vi "BGK Data Acquisition Loop - NLHQ.vi"(7 "Period (s)":dbl=600.0 caption="采样周期 (s)" format="%#_13g", 8 "error in (no error)":errorcluster caption="错误输入（无错误）", 11 "Message Queues":T1 caption="消息队列") -> (0 "error out":errorcluster caption="错误输出")   [LabVIEW 2015]
uses:
  Support VIs/Message Queue/All Real-Time Message Queues.ctl
  Support VIs/Message Queue/Message Cluster.ctl
  <vilib>/Platform/TimedLoop/XDataNode/timing_clust.ctl
  <vilib>/Platform/TimedLoop/XDataNode/nitl_modes.ctl
  <vilib>/Platform/TimedLoop/XDataNode/wakeup.ctl
  <vilib>/Instr/_visa.llb/VISA Configure Serial Port (Instr).vi
  Globals/Global - Monitoring Variables.vi
  <vilib>/Platform/TimedLoop/XDataNode/loadnilvce.vi
  Globals/Global - All RT Loop Stop.vi
  <vilib>/Platform/TimedLoop/XDataNode/XDataNode.xnode
  <vilib>/Platform/TimedLoop/XDataNode/XDNodeRunTimeDep.lvlib
  Support VIs/Message Queue/Message Queue.lvlib
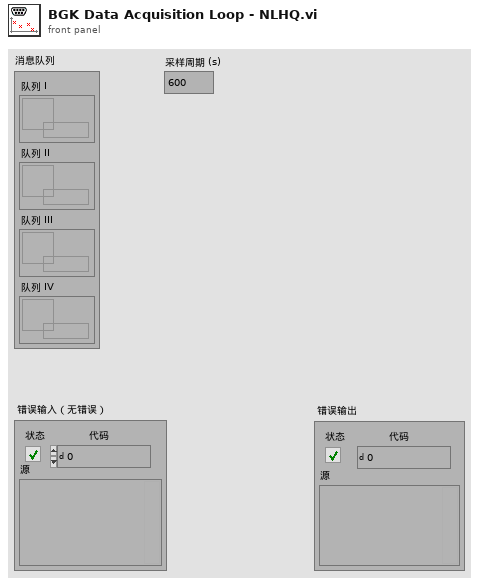
[diagram p1: front panel]
types:
  T1 = typedef "Message Queue.lvlib/All Real-Time Message Queues.ctl" = cluster{"Queue I":refnum<queue>, "Queue II":refnum<queue>, "Queue III":refnum<queue>, "Queue IV":refnum<queue>}
  T2 = typedef "XDNodeRunTimeDep.lvlib/timing_clust.ctl" = cluster{"Expected End [f-1]":u64, "Actual End [f-1]":u64, "Finished Late? [f-1]":bool, "Expected End [i-1]":u64, "Actual End [i-1]":u64, "Finished Late? [i-1]":bool, "Expected Start [i]":u64, "Actual Start [i]":u64, "Expected Start [f]":u64, "Actual Start [f]":u64, "Source Name":string, "Structure Name":string, "Period":i64, "Deadline":i64, "Offset":i64, "Start":i64, "Priority":i32, "Timeout":i32, "Mode":T3, "Wakeup Reason":T4, "Error":errorcluster, "Source Type":string, "Secondary Source Type":string, "Global End Time":u64, "Global Start Time":u64, "Frame Duration":u64, "Iteration Duration":u64, "Assigned CPU":i32, "I/O Scan Engine Mode":u32}
  T3 = typedef "XDNodeRunTimeDep.lvlib/nitl_modes.ctl" = enum32{"No Change", "Process missed periods, maintain original phase", "Discard missed periods, maintain original phase", "Process missed periods, ignore original phase", "Discard missed periods, ignore original phase"}
  T4 = typedef "XDNodeRunTimeDep.lvlib/wakeup.ctl" = enum32{"Normal", "Aborted", "Asynchronous wakeup", "Timing source error", "Timed loop error", "Timeout"}
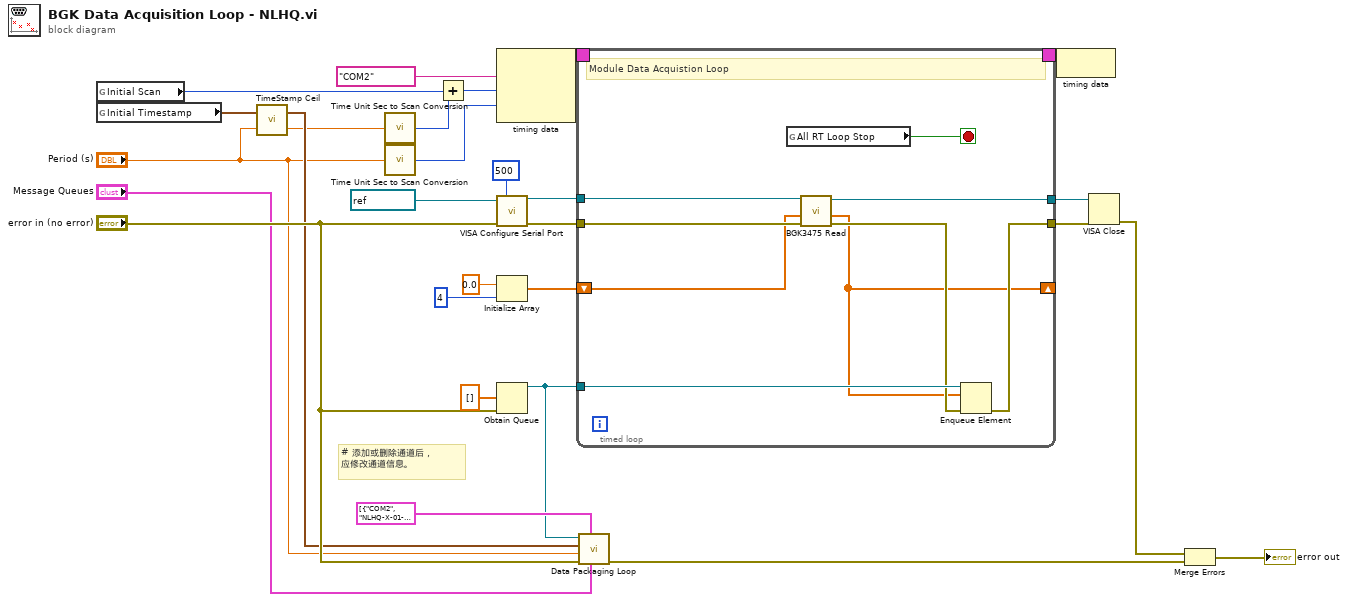
[diagram p0: block diagram]
diagram:
  # "# 添加或删除通道后，\n应修改通道信息。"
  n1 = global read "Global - Monitoring Variables.vi" "Initial Scan"() -> (w14:i64)
  n2 = global read "Global - Monitoring Variables.vi" "Initial Timestamp"() -> (w15:timestamp)
  n3 = call "TimeStamp Ceil.vi"("base (s)"="Period (s)", "timestamp input"=w15) -> ("time diff (s)"=w1:dbl, "timestamp output"=w7:timestamp)
  n4 = call "Time Unit Sec to Scan Conversion.vi"("time duration (s)"=w1) -> ("time duration (scan)"=w13:i64)
  n5 = call "Time Unit Sec to Scan Conversion.vi"("time duration (s)"="Period (s)") -> ("time duration (scan)"=w11:i64)
  n6 = Add(x=w14, y=w13) -> (x+y=w12:i64)
  n7 = node-c288("COM2" ("Structure Name"), w12, w11) -> (w27:T2)
  n8 = call-poly "VISA Configure Serial Port"("VISA resource name"=refnum<visa-resource-name> "COM2", "timeout (10sec)"=u32 500, "error in (no error)"="error in (no error)") -> ("VISA resource name out"=w20:refnum<visa-resource-name>, "error out"=w24:errorcluster)  [unwired: 11 in]
  n9 = Initialize Array(0.0 ("元素"), 4 ("维数大小")) -> (w3:dbl[])
  n10 = Obtain Queue(element data type=dbl[] [] ("数据类型"), error in (no error)="error in (no error)") -> (queue out=w8:refnum<queue>)  [unwired: 3 in, 2 out]
  n11 = timed-loop {
    timing: w27 -> [_]
    timing-out: [_] -> w26
    tunnel: w8 -> [w36]
    tunnel: w24 -> [w31]
    tunnel: [w35] -> w22
    tunnel: [w34] -> w23
    tunnel: w20 -> [w32]
    shift-right: [w29] -> _
    shift-left: w3 -> [w30]
    stop <- w37 stop-if-true
    # "Module Data Acquistion Loop"
    n12 = global read "Global - All RT Loop Stop.vi" "All RT Loop Stop"() -> (w37:bool)
    n13 = call "BGK3475 Read.vi"("error in (no error)"=w31, "Last Data Array"=w30, "VISA Ref Input"=w32) -> ("error out"=w33:errorcluster, "New Data Array"=w29:dbl[], "VISA Ref Output"=w34:refnum<visa-resource-name>)  [unwired: 6 in]
    n14 = Enqueue Element(queue=w36, element=w29, error in (no error)=w33) -> (error out=w35:errorcluster)  [unwired: 1 in, 2 out]
  }
  n15 = call "Data Packaging Loop.vi"("Message Queues"="Message Queues", "channel info array"=cluster{"Module":string, "Channel":string}[] [{"Module"="COM2", "Channel"="NLHQ-X-01-D01"}, {"Module"="COM2", "Channel"="NLHQ-X-02-D01"}, {"Module"="COM2", "Channel"="NLHQ-X-04-D01"}, {"Module"="COM2", "Channel"="NLHQ-X-06-D01"}], "error in (no error)"="error in (no error)", "sampling period (s)"="Period (s)", "timestamp"=w7, "data queue"=w8) -> ("error out"=w16:errorcluster)  [unwired: 5 in]
  n16 = node-c288(w26) -> ()
  n17 = VISA Close(VISA resource name=w23, error in (no error)=w22) -> (error out=w21:errorcluster)
  n18 = Merge Errors(w21, w16) -> (→"error out":errorcluster)
